vi "RGB to HSL.vi"(10 "Destination (HSL)":T1, 11 "Image (RGB)":T1) -> (3 "Image Out (HSL)":T1)   [LabVIEW 2012]
uses:
  <vilib>/vision/Image Controls.llb/IMAQ Image.ctl
  <vilib>/vision/NI_Vision_Development_Module.lvlib
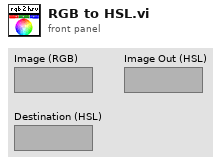
[diagram p1: front panel]
types:
  T1 = typedef "IMAQ Image.ctl" = refnum<image>
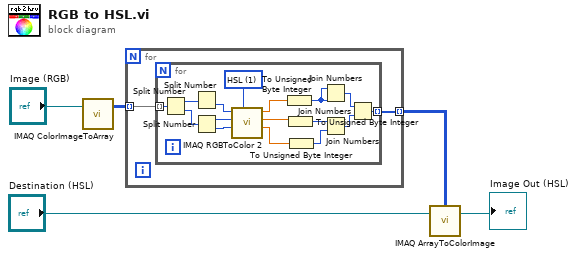
[diagram p0: block diagram]
diagram:
  n1 = call "IMAQ ColorImageToArray"("Image"="Image (RGB)") -> ("Image Pixels (U32)"=w2:u32[][])  [unwired: 3 in, 2 out]
  n2 = for {
    tunnel: w2 -> [w7] mode=indexing
    tunnel: [w6] -> w3 mode=indexing
    n3 = for {
      tunnel: w7 -> [w23] mode=indexing
      tunnel: [w8] -> w6 mode=indexing
      w20 = u16 1 items=["RGB", "HSL", "HSV", "HSI", "CIE L*a*b*", "CIE XYZ"] ("Color Mode")
      n4 = Split Number(x=w23) -> (hi(x)=w22:u16, lo(x)=w21:u16)
      n5 = Split Number(x=w22) -> (lo(x)=w19:u8)  [unwired: 1 out]
      n6 = Split Number(x=w21) -> (hi(x)=w18:u8, lo(x)=w17:u8)
      n7 = call "IMAQ RGBToColor 2"("Color Mode"=w20, "Blue value"=w17, "Green value"=w18, "Red value"=w19) -> ("Blue or Luma or Val or Inten or Z or b*value"=w14:dbl, "Green or Sat or Y or a* value"=w15:dbl, "Red or Hue or X or L* value"=w16:dbl)  [unwired: 4 in, 1 out]
      n8 = To Unsigned Byte Integer(number=w16) -> (unsigned 8bit integer=w13:u8)
      n9 = To Unsigned Byte Integer(number=w15) -> (unsigned 8bit integer=w12:u8)
      n10 = To Unsigned Byte Integer(number=w14) -> (unsigned 8bit integer=w11:u8)
      n11 = Join Numbers(hi=w13, lo=w13) -> ((hi.lo)=w10:u16)
      n12 = Join Numbers(hi=w12, lo=w11) -> ((hi.lo)=w9:u16)
      n13 = Join Numbers(hi=w10, lo=w9) -> ((hi.lo)=w8:u32)
    }
  }
  n14 = call "IMAQ ArrayToColorImage"("Image Pixels (U32)"=w3, "Image"="Destination (HSL)") -> ("Image Out"=→"Image Out (HSL)":T1)  [unwired: 3 in, 1 out]
